vi "motpar1.vi"() -> (3 "w":dbl)   [LabVIEW 2015]
panel:
  in  "ke":dbl=0.26
  in  "kt":dbl=0.26
  in  "t":dbl=1.36
  in  "r":dbl=0.5
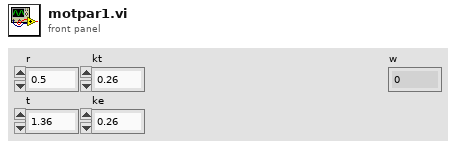
[diagram p1: front panel]
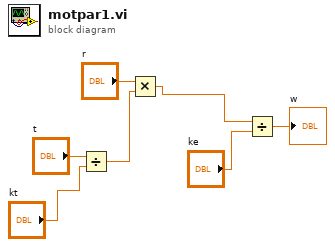
[diagram p0: block diagram]
diagram:
  n1 = Divide(x="t", y="kt") -> (x/y=w6:dbl)
  n2 = Multiply(x="r", y=w6) -> (x*y=w3:dbl)
  n3 = Divide(x=w3, y="ke") -> (x/y=→"w":dbl)
